vi "SIM_PositionOutput.vi"(9 "array":dbl[][](array[numeric]), 10 "Position (Reframed)":cluster{"x (m)":dbl, "y (m)":dbl, "z (mm)":dbl} {"z (mm)" format="%.1f"; "y (m)" format="%.1p"; "x (m)" format="%.1p"}) -> (2 "Signal Out":dbl, 4 "Zread":dbl, 6 "z (mm)":dbl)   [LabVIEW 2023]
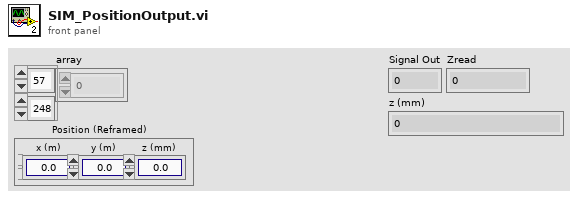
[diagram p1: front panel]
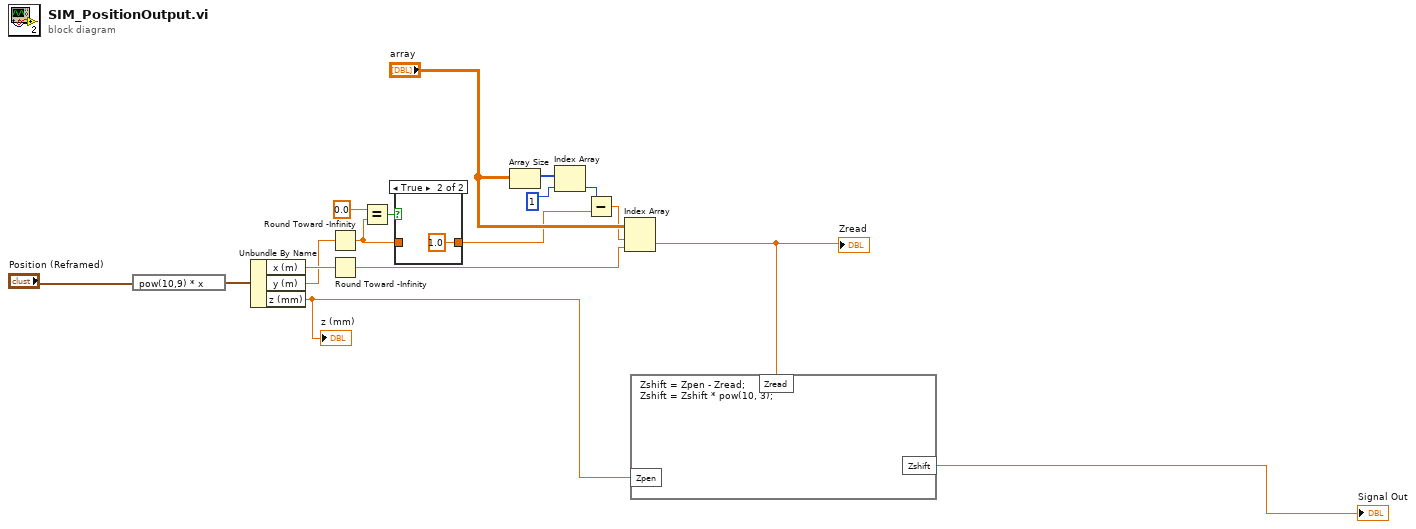
[diagram p0: block diagram]
diagram:
  n1 = expression code="pow(10,9) * x"("Position (Reframed)") -> (w15:cluster{"x (m)":dbl, "y (m)":dbl, "z (mm)":dbl})
  n2 = Unbundle By Name(w15) -> ("x (m)"=w14:dbl, "y (m)"=w13:dbl, "z (mm)"=w2:dbl)
  "z (mm)" <- w2
  n3 = Round Toward -Infinity(1:w13) -> (0:w4:dbl)
  n4 = Round Toward -Infinity(1:w14) -> (0:w17:dbl)
  n5 = Equal?(x=0.0, y=w4) -> (x = y?=w7:bool)
  n6 = case shown="True" w7 {
    tunnel: [w18 1.0] -> w5
    tunnel: w4 -> [w18 _]
    frame False {
    }
    frame True {
    }
  }
  n7 = Array Size(array="array") -> (size(s)=w11:i32[])
  n8 = Index Array(array=w11, index=1) -> (element=w8:i32)
  n9 = Subtract(x=w8, y=w5) -> (x-y=w9:dbl)
  n10 = Index Array(array="array", index (row)=w9, index (col)=w17) -> (element=w3:dbl)
  "Zread" <- w3
  n11 = formula code="Zshift = Zpen - Zread;\nZshift = Zshift * pow(10, 3);"("Zread"=w3, "Zpen"=w2) -> ("Zshift"=→"Signal Out":dbl)
